vi "Update LimitCurrent Attribute.vi"(8 "error in":errorcluster, 10 "Scale From Config Max":dbl format="%.7f", 11 "PS Driver in":refnum<class "PS Driver.lvclass">) -> (0 "error out":errorcluster, 2 "Variant":variant, 3 "PS Driver out":refnum<class "PS Driver.lvclass">)   [LabVIEW 2024, in "PS Driver.lvlib" / "PS Driver.lvclass"]
uses:
  PS Driver.lvclass
  PS Driver.lvclass/PS Driver.ctl
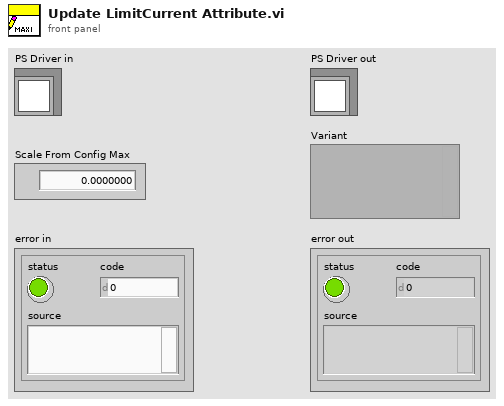
[diagram p1: front panel]
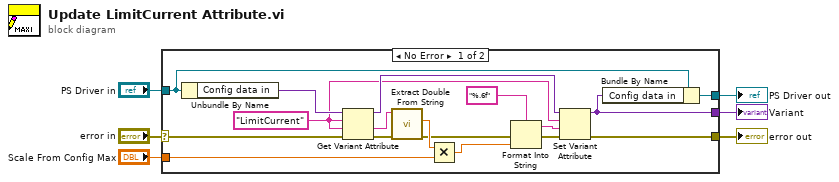
[diagram p0: block diagram]
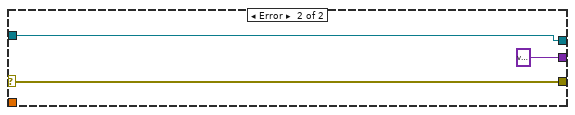
[diagram p2: hidden frame]
diagram:
  n1 = case shown="No Error" "error in" {
    selector: "error in" -> [w18 w25]
    tunnel: [w8 w25] -> w5
    tunnel: [w23 w26] -> w3
    tunnel: "PS Driver in" -> [w22 w26]
    tunnel: "Scale From Config Max" -> [w16 _]
    tunnel: [w7 variant] -> w1
    frame No Error {
      w12 = "LimitCurrent" ("name")
      n2 = Unbundle By Name(w22) -> ("Config data in"=w19:variant)
      n3 = Get Variant Attribute(Variant=w19, name=w12, default value (empty Variant)=w12, error in=w18) -> (duplicate Variant=w13:variant, value=w21:string, error out=w20:errorcluster)  [unwired: 1 out]
      n4 = call "Extract Double From String.vi"("error in"=w20, "string"=w21) -> ("error out"=w9:errorcluster, "floating pt. number"=w17:dbl)  [unwired: 2 in, 2 out]
      n5 = Multiply(x=w17, y=w16) -> (x*y=w15:dbl)
      n6 = Format Into String(format string="%.6f", error in=w9, w15) -> (resulting string=w11:string, error out=w10:errorcluster)  [unwired: 1 in]
      n7 = Set Variant Attribute(Variant=w13, name=w12, value=w11, error in=w10) -> (Variant out=w7:variant, error out=w8:errorcluster)  [unwired: 1 out]
      n8 = Bundle By Name(cluster=w22, "Config data in"=w7) -> (w23:refnum<class "PS Driver.lvclass">)
    }
    frame Error {
    }
  }
  "error out" <- w5
  "PS Driver out" <- w3
  "Variant" <- w1
